vi "ReadVI.vi"(7 "Enum":T1, 8 "error in (no error)":errorcluster, 9 "Param in":T2, 10 "queue in":refnum<queue>) -> (0 "error out":errorcluster)   [LabVIEW 2023]
uses:
  Param out.ctl
  enum_readfile_loop.ctl
  enum_FGV.ctl
  Param in.ctl
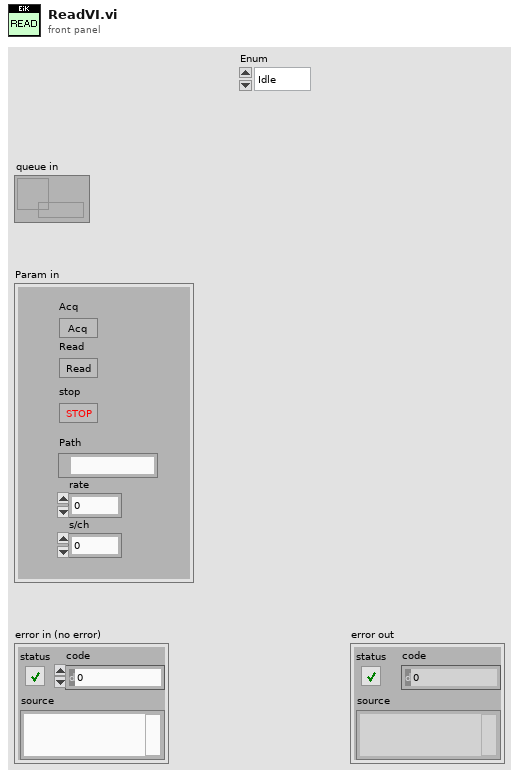
[diagram p1: front panel]
types:
  T1 = typedef "enum_readfile_loop.ctl" = enum16{"Idle", "Initialize", "Read_file", "End"}
  T2 = typedef "Param out.ctl" = cluster{"Acq":bool, "stop":bool, "Path":path, "rate":dbl, "s/ch":dbl, "Read":bool}
  T3 = typedef "enum_FGV.ctl" = enum16{"Get", "Set"}
  T4 = enum16{"open", "open or create", "create or replace", "create", "open (read-only)"}
  T5 = typedef "Param in.ctl" = cluster{"Acq":bool, "stop":bool, "Path":path, "rate":dbl, "s/ch":dbl, "Read":bool}
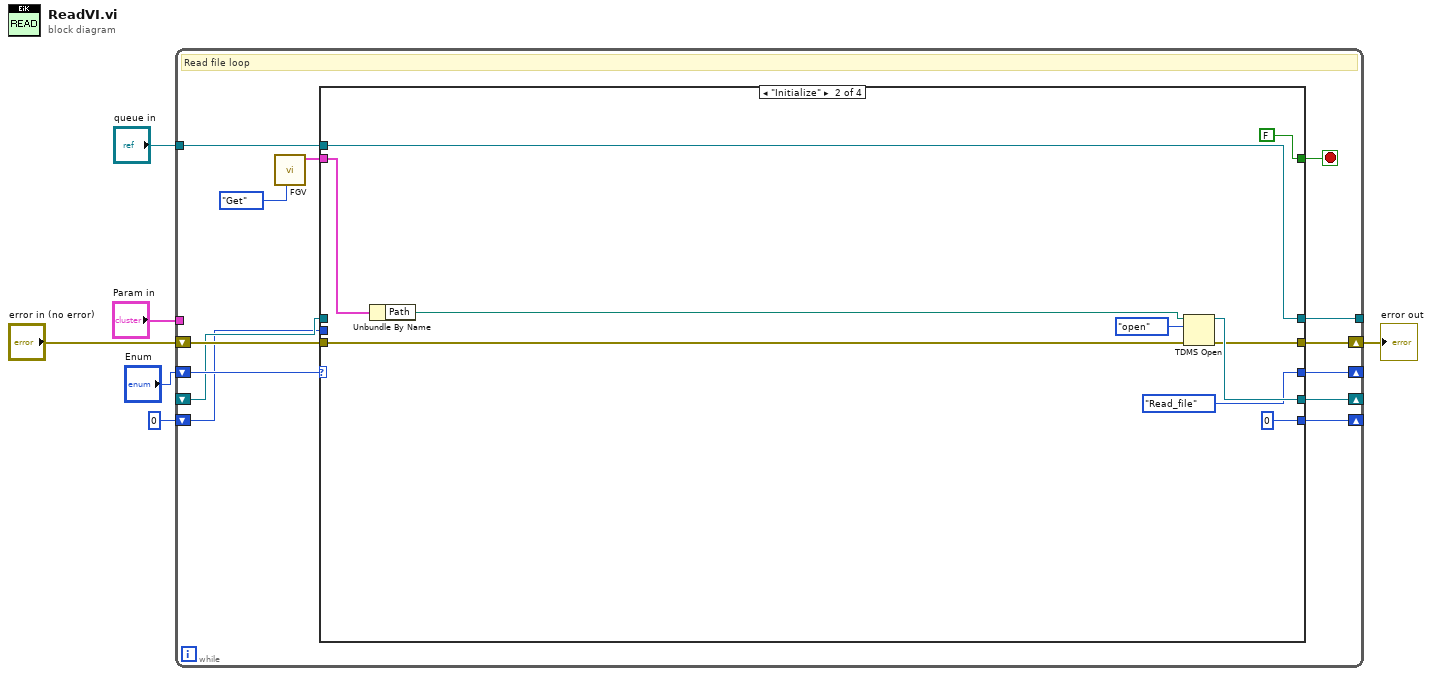
[diagram p0: block diagram]
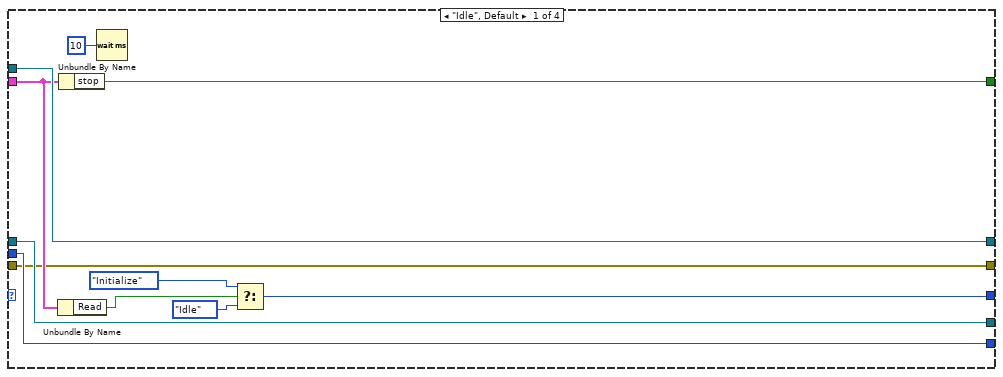
[diagram p2: hidden frame]
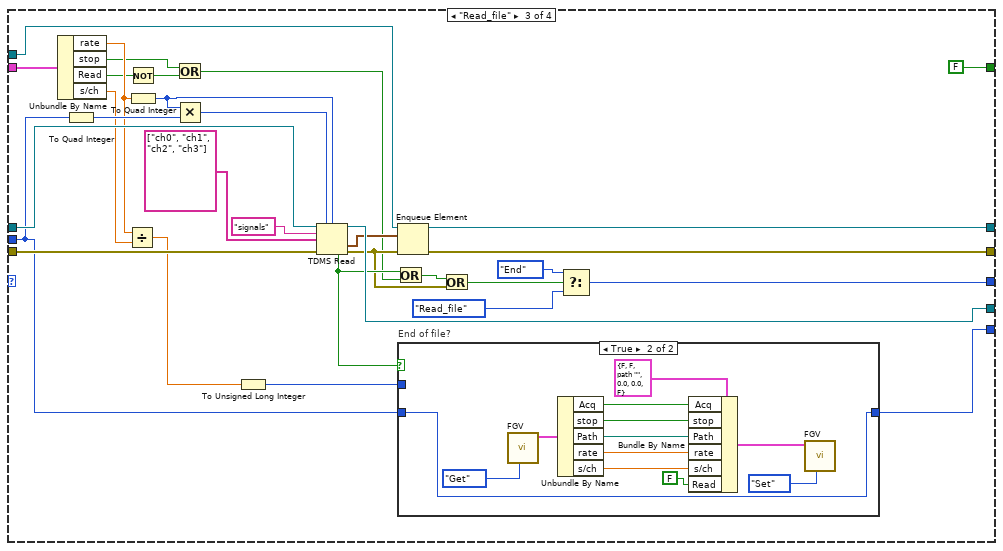
[diagram p3: hidden frame]
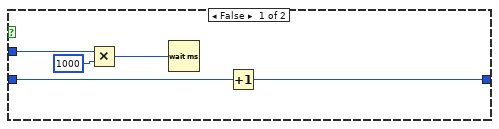
[diagram p4: hidden frame]
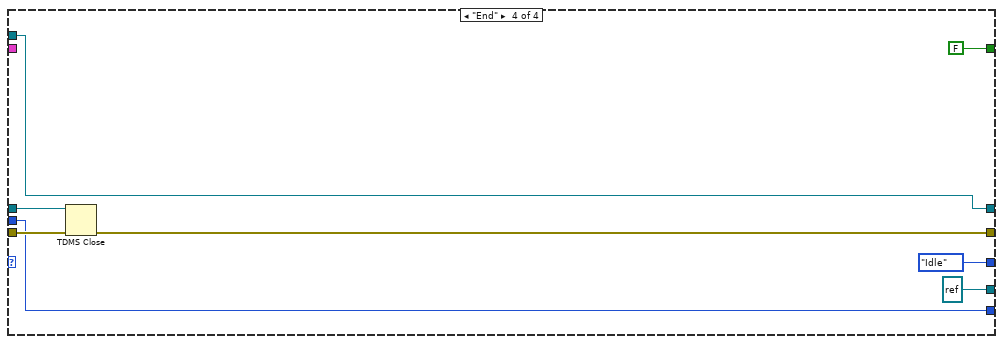
[diagram p5: hidden frame]
diagram:
  n1 = while {
    shift-right: [w18] -> _
    shift-left: "Enum" -> [w19]
    shift-right: [w10] -> w3
    shift-left: "error in (no error)" -> [w17]
    shift-right: [w16] -> _
    shift-left: _ -> [w15]
    shift-right: [w13] -> _
    shift-left: 0 -> [w14]
    tunnel: "queue in" -> [w12]
    tunnel: [w11] -> _
    tunnel: "Param in" -> [_]
    stop <- w7 stop-if-true
    # "Read file loop"
    n2 = call "FGV.vi"("Action"=enum_FGV."Get") -> ("Param out"=w9:T2)  [unwired: 10 in]
    n3 = case shown="\"Initialize\"" w19 {
      tunnel: [w27 enum_readfile_loop."Read_file" w56 enum_readfile_loop."Idle"] -> w18
      tunnel: w17 -> [w20 w39 w68 w95]
      tunnel: [w20 w31 w59 w94] -> w10
      tunnel: [w26 w38 w69 refnum<k34> refnum ("tdms file")] -> w16
      tunnel: w15 -> [w26 _ w70 w96]
      tunnel: w14 -> [w25 _ w65 w92]
      tunnel: [w25 0 w71 w92] -> w13
      tunnel: w12 -> [w24 w36 w61 w90]
      tunnel: [w24 w36 w60 w90] -> w11
      tunnel: w9 -> [w22 w35 w55 _]
      tunnel: [w21 FALSE ("stop") FALSE ("stop") FALSE ("stop")] -> w7
      frame "Idle", Default {
        n4 = Unbundle By Name(w22) -> ("Read"=w23:bool)
        n5 = Unbundle By Name(w22) -> ("stop"=w21:bool)
        n6 = Wait (ms)(milliseconds to wait=u32 10) -> ()  [unwired: 1 out]
        n7 = Select(t=enum_readfile_loop."Initialize", s=w23, f=enum_readfile_loop."Idle") -> (s? t:f=w27:T1)
      }
      frame "Initialize" {
        n8 = Unbundle By Name(w35) -> ("Path"=w34:path)
        n9 = TDMS Open(8:w39, 10:T4."open" ("operation (0:open)"), 11:w34) -> (0:w31:errorcluster, 3:w38:refnum<k34>)  [unwired: 4 in]
      }
      frame "Read_file" {
        n10 = Unbundle By Name(w55) -> ("rate"=w51:dbl, "stop"=w42:bool, "Read"=w43:bool, "s/ch"=w45:dbl)
        n11 = To Quad Integer(1:w65) -> (0:w64:i64)
        n12 = Divide(x=w51, y=w45) -> (x/y=w49:dbl)
        n13 = Not(x=w43) -> (.not. x?=w44:bool)
        n14 = To Quad Integer(1:w51) -> (0:w52:i64)
        n15 = Or(x=w42, y=w44) -> (x .or. y?=w41:bool)
        n16 = Multiply(x=w52, y=w64) -> (x*y=w63:i64)
        n17 = To Unsigned Long Integer(number=w49) -> (unsigned 32bit integer=w50:u32)
        n18 = TDMS Read(0:w70, 1:w63, 2:w52, 5:"signals" ("group name in"), 7:string[] ["ch0", "ch1", "ch2", "ch3"] ("channel name(s) in"), 11:w68) -> (4:w69:refnum<k34>, 10:w62:waveform(dbl)[], 14:w53:bool, 15:w46:errorcluster)  [unwired: 2 in, 2 out]
        n19 = Or(x=w53, y=w41) -> (x .or. y?=w47:bool)
        n20 = Enqueue Element(queue=w61, element=w62, error in (no error)=w46) -> (queue out=w60:refnum<queue>, error out=w59:errorcluster)  [unwired: 1 in, 1 out]
        n21 = case "End of file?" shown="True" w53 {
          tunnel: w65 -> [w76 w88]
          tunnel: [w75 w88] -> w71
          tunnel: w50 -> [w72 _]
          frame False {
            # "End of file?"
            n22 = Multiply(x=w72, y=u32 1000 ("milliseconds to wait")) -> (x*y=w74:u32)
            n23 = Wait (ms)(milliseconds to wait=w74) -> ()  [unwired: 1 out]
            n24 = Increment(x=w76) -> (x+1=w75:i32)
          }
          frame True {
            # "End of file?"
            n25 = call "FGV.vi"("Action"=enum_FGV."Get") -> ("Param out"=w86:T2)  [unwired: 10 in]
            n26 = Unbundle By Name(w86) -> ("Acq"=w85:bool, "stop"=w84:bool, "Path"=w83:path, "rate"=w82:dbl, "s/ch"=w81:dbl)
            n27 = Bundle By Name(cluster=T5 {"Acq"=FALSE, "stop"=FALSE, "Path"=path "", "rate"=0.0, "s/ch"=0.0, "Read"=FALSE} ("Param in"), "Acq"=w85, "stop"=w84, "Path"=w83, "rate"=w82, "s/ch"=w81, "Read"=FALSE) -> (w79:T5)
            n28 = call "FGV.vi"("Action"=enum_FGV."Set", "Param in"=w79) -> ()  [unwired: 9 in, 1 out]
          }
        }
        n29 = Or(x=w47, y=w46) -> (x .or. y?=w48:bool)
        n30 = Select(t=enum_readfile_loop."End", s=w48, f=enum_readfile_loop."Read_file") -> (s? t:f=w56:T1)
      }
      frame "End" {
        n31 = TDMS Close(8:w95, 11:w96) -> (0:w94:errorcluster)  [unwired: 1 out]
      }
    }
  }
  "error out" <- w3
